vi "StartStopConversion.vi"(8 "error in (no error)":errorcluster, 11 "Model Driver in":refnum<class "Model Driver.lvclass">) -> (0 "error out":errorcluster, 3 "Model Driver out":refnum<class "Model Driver.lvclass">)   [LabVIEW 2023, in "Model Driver.lvclass"]
doc: "This method starts/stops the ADC convertion VI when Start/stop is pressed."
uses:
  Model Driver.lvclass
  Type def/variant.ctl
  Type def/QueueOperations.ctl
  Model Driver.lvclass/Model Driver.ctl
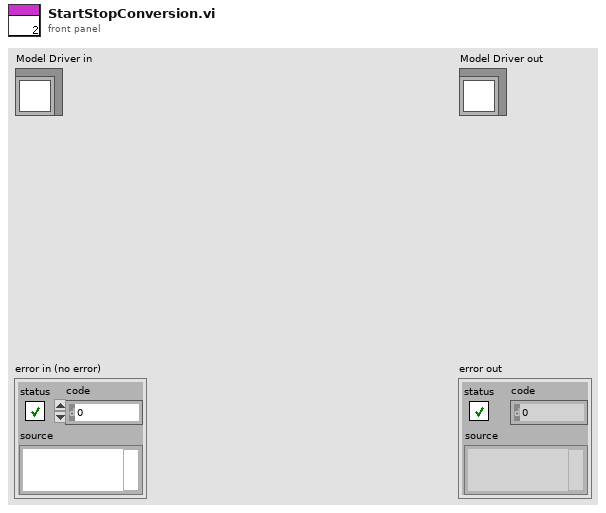
[diagram p1: front panel]
types:
  T1 = typedef "QueueOperations.ctl" = enum16{"Create", "Enqueue", "Enqueue N elements", "Dequeue", "Flush", "Release"}
  T2 = typedef "variant.ctl" = cluster{"Data":variant, "State":string}
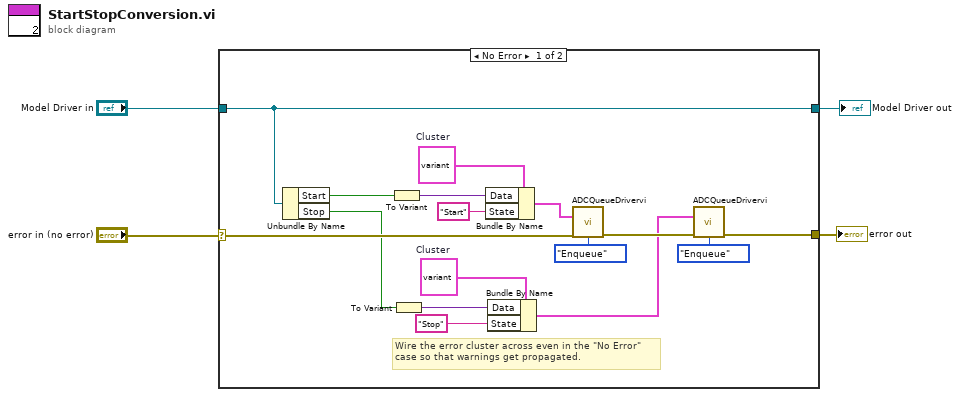
[diagram p0: block diagram]
diagram:
  n1 = case shown="No Error" "error in (no error)" {
    selector: "error in (no error)" -> [w9 w22]
    tunnel: [w8 w22] -> w3
    tunnel: [w7 w21] -> w1
    tunnel: "Model Driver in" -> [w7 w21]
    frame No Error {
      w14 = T2 {"Data"=variant, "State"=""}  # Cluster
      w19 = T2 {"Data"=variant, "State"=""}  # Cluster
      # "Wire the error cluster across even in the \"No Error\"\ncase so that warnings get propagated."
      n2 = Unbundle By Name(w7) -> ("Start"=w6:bool, "Stop"=w5:bool)
      n3 = To Variant(anything=w6) -> (Variant=w18:variant)
      n4 = To Variant(anything=w5) -> (Variant=w15:variant)
      n5 = Bundle By Name(cluster=w19, "Data"=w18, "State"="Start") -> (w16:T2)
      n6 = Bundle By Name(cluster=w14, "Data"=w15, "State"="Stop") -> (w11:T2)
      n7 = call "ADCQueueDrivervi.vi"("Enqueue State"=w16, "error in"=w9, "Queue Operations"=QueueOperations."Enqueue") -> ("error out"=w12:errorcluster)  [unwired: 11 in, 1 out]
      n8 = call "ADCQueueDrivervi.vi"("Enqueue State"=w11, "error in"=w12, "Queue Operations"=QueueOperations."Enqueue") -> ("error out"=w8:errorcluster)  [unwired: 11 in, 1 out]
    }
    frame Error {
    }
  }
  "error out" <- w3
  "Model Driver out" <- w1
